vi "InWindow_Reach.vi"(1 "TargetsCluster":T2 {"Pos8"."Radius" min=-5.0 max=5.0 step=0.5 format="%.2f"; "Pos8"."Vert" min=-5.0 max=5.0 step=0.5 format="%.2f"; "Pos8"."Horiz" min=-5.0 max=5.0 step=0.5 format="%.2f"; "Pos7"."Radius" min=-5.0 max=5.0 step=0.5 format="%.2f"; "Pos7"."Vert" min=-5.0 max=5.0 step=0.5 format="%.2f"; "Pos7"."Horiz" min=-5.0 max=5.0 step=0.5 format="%.2f"; "Pos6"."Radius" min=-5.0 max=5.0 step=0.5 format="%.2f"; "Pos6"."Vert" min=-5.0 max=5.0 step=0.5 format="%.2f"; "Pos6"."Horiz" min=-5.0 max=5.0 step=0.5 format="%.2f"; "Pos5"."Radius" min=-5.0 max=5.0 step=0.5 format="%.2f"; "Pos5"."Vert" min=-5.0 max=5.0 step=0.5 format="%.2f"; "Pos5"."Horiz" min=-5.0 max=5.0 step=0.5 format="%.2f"; "Pos4"."Radius" min=-5.0 max=5.0 step=0.5 format="%.2f"; "Pos4"."Vert" min=-5.0 max=5.0 step=0.5 format="%.2f"; "Pos4"."Horiz" min=-5.0 max=5.0 step=0.5 format="%.2f"; "Pos3"."Radius" min=-5.0 max=5.0 step=0.5 format="%.2f"; "Pos3"."Vert" min=-5.0 max=5.0 step=0.5 format="%.2f"; "Pos3"."Horiz" min=-5.0 max=5.0 step=0.5 format="%.2f"; "Pos2"."Radius" min=-5.0 max=5.0 step=0.5 format="%.2f"; "Pos2"."Vert" min=-5.0 max=5.0 step=0.5 format="%.2f"; "Pos2"."Horiz" min=-5.0 max=5.0 step=0.5 format="%.2f"; "Pos1"."Radius" min=-5.0 max=5.0 step=0.5 format="%.2f"; "Pos1"."Vert" min=-5.0 max=5.0 step=0.5 format="%.2f"; "Pos1"."Horiz" min=-5.0 max=5.0 step=0.5 format="%.2f"; "Start"."Radius" min=-5.0 max=5.0 step=0.5 format="%.2f"; "Start"."Vert" min=-5.0 max=5.0 step=0.5 format="%.2f"; "Start"."Horiz" min=-5.0 max=5.0 step=0.5 format="%.2f"}, 2 "xyArray":dbl[](array[numeric])) -> (0 "StatusCluster":T1)   [LabVIEW 2011]
uses:
  <vilib>/imath/engines/lvmath2/RunTimeEngine/ErrorHandling/NIMS_Finalize Error.vi
  <vilib>/imath/engines/lvmath2/RunTimeEngine/NodeEndStatement/NIMS_NodeEndStatement_Output.vi
  <instcachedir>/0/NIMS_NodeEndStatement_Output_53EC0D466D134D7ABD903AC30B43404B.lvgen/NIMS_NodeEndStatement_Output_53EC0D466D134D7ABD903AC30B43404B_011.vi
  <vilib>/imath/engines/lvmath2/RunTimeEngine/RangeToken/NIMS_Range_R2.vi
  <vilib>/imath/engines/lvmath2/RunTimeEngine/BuiltInFunctions/size/NIMS_I32=size(GM,I32).vi
  <instcachedir>/0/NIMS_I32=size(GM,I32)_C888250C35F946008B07D98778967D76.lvgen/NIMS_I32=size(GM,I32)_C888250C35F946008B07D98778967D76_004.vi
  <vilib>/imath/engines/lvmath2/RunTimeEngine/VariableToken/Read/NIMS_Get Elements - SorM($,_) - Check.vi
  <instcachedir>/0/NIMS_Get Elements - SorM($,_) - Check_5DE9D7AB93274078B6FA87EFB9C11DB1.lvgen/NIMS_Get Elements - SorM($,_) - Check_5DE9D7AB93274078B6FA87EFB9C11DB1_003.vi
  <vilib>/imath/engines/lvmath2/RunTimeEngine/BuiltInFunctions/repeatmx/NIMS_repeatmx(GM, I32, I32).vi
  <instcachedir>/0/NIMS_repeatmx(GM, I32, I32)_8C2ED2EBCBCE41FC8E83AC0E124C0986.lvgen/NIMS_repeatmx(GM, I32, I32)_8C2ED2EBCBCE41FC8E83AC0E124C0986_000.vi
  <vilib>/imath/engines/lvmath2/RunTimeEngine/ArithmeticOperatorToken/NIMS_ArithmeticOperator_minus.vi
  <instcachedir>/0/NIMS_ArithmeticOperator_minus_27860A2576AF4B729B9D72749D8AAD88.lvgen/NIMS_ArithmeticOperator_minus_27860A2576AF4B729B9D72749D8AAD88_002.vi
  <vilib>/imath/engines/lvmath2/RunTimeEngine/BuiltInFunctions/sum/NIMS_sum(GM,Sca).vi
  <instcachedir>/0/NIMS_sum(GM,Sca)_ABC1F592A4F346FDB139C97B43B4EE64.lvgen/NIMS_sum(GM,Sca)_ABC1F592A4F346FDB139C97B43B4EE64_001.vi
  <vilib>/imath/engines/lvmath2/RunTimeEngine/ErrorHandling/NIMS_Create Error From Enums.vi
  <instcachedir>/0/NIMS_Get Elements - SorM($,_) - Check_5DE9D7AB93274078B6FA87EFB9C11DB1.lvgen/NIMS_Get Elements - SorM($,_) - Check_5DE9D7AB93274078B6FA87EFB9C11DB1_000.vi
  <vilib>/imath/engines/lvmath2/RunTimeEngine/RelationalOperatorToken/NIMS_Relational_Operator_Le.vi
  <instcachedir>/0/NIMS_Relational_Operator_Le_1AD62C9870854D23918503CE42CF56F4.lvgen/NIMS_Relational_Operator_Le_1AD62C9870854D23918503CE42CF56F4_004.vi
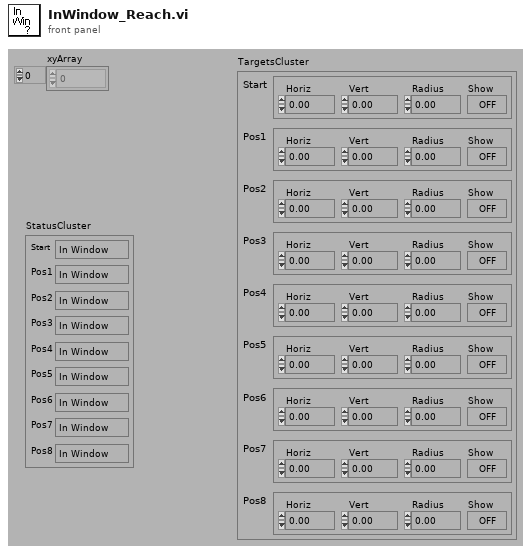
[diagram p1: front panel]
types:
  T1 = cluster{"Start":enum16{"In Window", "Out Window"}, "Pos1":enum16{"In Window", "Out Window"}, "Pos2":enum16{"In Window", "Out Window"}, "Pos3":enum16{"In Window", "Out Window"}, "Pos4":enum16{"In Window", "Out Window"}, "Pos5":enum16{"In Window", "Out Window"}, "Pos6":enum16{"In Window", "Out Window"}, "Pos7":enum16{"In Window", "Out Window"}, "Pos8":enum16{"In Window", "Out Window"}}
  T2 = cluster{"Start":cluster{"Horiz":dbl, "Vert":dbl, "Radius":dbl, "Show":bool}, "Pos1":cluster{"Horiz":dbl, "Vert":dbl, "Radius":dbl, "Show":bool}, "Pos2":cluster{"Horiz":dbl, "Vert":dbl, "Radius":dbl, "Show":bool}, "Pos3":cluster{"Horiz":dbl, "Vert":dbl, "Radius":dbl, "Show":bool}, "Pos4":cluster{"Horiz":dbl, "Vert":dbl, "Radius":dbl, "Show":bool}, "Pos5":cluster{"Horiz":dbl, "Vert":dbl, "Radius":dbl, "Show":bool}, "Pos6":cluster{"Horiz":dbl, "Vert":dbl, "Radius":dbl, "Show":bool}, "Pos7":cluster{"Horiz":dbl, "Vert":dbl, "Radius":dbl, "Show":bool}, "Pos8":cluster{"Horiz":dbl, "Vert":dbl, "Radius":dbl, "Show":bool}}
  T3 = cluster{"Horiz":dbl, "Vert":dbl, "Radius":dbl, "Show":bool}[]
  T4 = cluster{"[0]":i16, "[1]":i16, "[2]":i16, "[3]":i16, "[4]":i16, "[5]":i16, "[6]":i16, "[7]":i16, "[8]":i16}
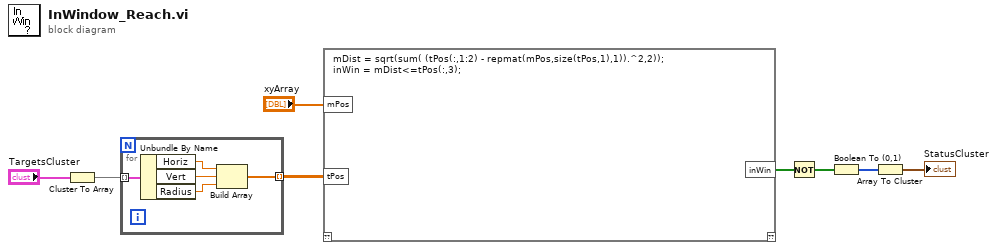
[diagram p0: block diagram]
diagram:
  n1 = Cluster To Array(cluster="TargetsCluster") -> (array=w3:T3)
  n2 = for {
    tunnel: w3 -> [w13] mode=indexing
    tunnel: [w9] -> w2 mode=indexing
    n3 = Unbundle By Name(w13) -> ("Horiz"=w11:dbl, "Vert"=w12:dbl, "Radius"=w10:dbl)
    n4 = Build Array(w11, w12, w10) -> (w9:dbl[])
  }
  n5 = mathscript code="mDist = sqrt(sum( (tPos(:,1:2) - repmat(mPos,size(tPos,1),1)).^2,2));\ninWin = mDist<=tPos(:,3);"("mPos"="xyArray", "tPos"=w2) -> ("inWin"=w6:bool[])  [unwired: 1 in, 1 out]
  n6 = Not(x=w6) -> (.not. x?=w5:bool[])
  n7 = Boolean To (0,1)(Boolean=w5) -> (0, 1=w8:i16[])
  n8 = Array To Cluster(array=w8) -> (cluster=→"StatusCluster":T4)
